vi "Demo.vi"() -> ()   [LabVIEW 2020, in "PowerControl.lvlib"]
uses:
  PowerControl.lvlib
  Labview Library/Libraries/Basic Experiment/CW settings.ctl
  YP03-60_X/YP03-60_X.lvclass
  C:/Labview Program/Labview_Control_SIC/Backup/VirtualPower/VirtualPower.lvclass
  YP03-60_Y/YP03-60_Y.lvclass
  YP03-60_Z/YP03-60_Z.lvclass
  VirtualPower/VirtualPower.lvclass
  Labview Library/Libraries/Basic Experiment/Basic Experiment.lvlib
panel:
  out "Pro":dbl[][](array[numeric])=[[-0.006013746913685614, -0.0005767508775091912, 0.003580211726197824, 0.002155800816019182, 0.0038511908961347263, 0.006438426694988175, -0.0017340280440567568, 0.005718743562201478, -0.004332868092551068, -0.00041017545622312745, -0.005538970864038539, -0.004012464200014998, -0.00792516643020258, -0.01574654474779913, -0.01310209587117428, -0.01651762842727922, -0.028081230793792877, -0.07887102008294333, -0.0966488744667412, -0.05726574286992636, -0.04009710278904244, -0.013943654119989213, -0.014891792267481052, -0.02856618593174698, -0.03385032526214127, -0.040599217504896146, -0.06044913845652411, -0.12219252863119912, -0.145572899201861, -0.12238330994007585, -0.07440755792421139, -0.04136503780617107, -0.03663431604289491, -0.022466284502222655, -0.009988690512261256, -0.007853472773907688, -0.0040597390725739535, -0.0010535701888517712, 0.001942673587738586, 0.0009046401382202252, -0.0022040602679889165], [0.00030942018483859357, 0.006545517163617287, -0.011571285455226787, -0.0005543704724179088, -0.00571613383603764, 0.003448168346978475, 0.0022478971389876534, -0.007040149065929868, 0.002513251653887716, 0.007368641761340111, 0.006313201433677307, -0.00947691386415117, -0.009153843171827547, -0.0012277679613130754, -0.009004290054349107, -0.022273516386379755, -0.04492940997686401, -0.07542469057166712, -0.10680439423841448, -0.06490179281471364, -0.043742806147826885, -0.03088586641820057, -0.03126158796986778, -0.03249904007682625, -0.04118533262413637, -0.06908010461555458, -0.10829568918119781, -0.1400238554264911, -0.10848703215017097, -0.06390484710798727, -0.03541632652309068, -0.019723273238761663, -0.017594711205418556, -0.01004862751091018, -0.00419887575862532, -0.011289191176208968, -0.003957013291320699, -0.00799541009422966, -0.005162780434214143, -0.006557950052931361, 0.00910905576244403], [0.006810636496503708, 0.010758157059567397, 0.00037187790202142246, -0.004975811124692475, -0.0022549265445015454, 0.004440990805914868, -0.005902149381657673, 0.0028450707010927445, -0.0013811589049794737, 0.005622914037517024, -0.007749721403714438, -0.011096664744028928, -0.006185456463094541, -0.014770720832796513, -0.006400699596351922, -0.01917068103315489, -0.03484291583179, -0.06696654295085125, -0.09429663190407978, -0.07022193366873686, -0.036127944880454343, -0.026433493814997933, -0.029596540512562775, -0.0547595204849165, -0.07934624397091083, -0.135303604851986, -0.14142779317873644, -0.11050981053166709, -0.05881398467255716, -0.042245426557882104, -0.02351994328283369, -0.019050385278118087, -0.009077854056939172, -0.007456997905022966, -0.004786728583101252, -0.01281291444557675, -0.0006758410166896045, -0.01320520210400744, 0.002038086253812299, 0.0057848989008100205, 0.0008845616357138208], [-0.002625712867039609, -0.0016672366841851138, 0.001523064957566156, 0.005031329580088562, 0.009562663666520255, -0.0133910818070474, 0.006351665826920705, -0.0032259111426599096, 0.002258900555879295, -0.001824194789903033, -0.010315416844289382, -0.014942445722062159, -0.010711646570336852, -0.008176873818602326, -0.0040919553812546194, -0.015920369318373595, -0.042856625587384456, -0.07552804437875049, -0.0974008995916611, -0.07697979712414382, -0.040526212336561174, -0.03947076513356085, -0.04879065588970799, -0.0785332509819675, -0.12130753027718966, -0.13003020401205556, -0.10267359275594912, -0.05305535890037516, -0.04023734109264043, -0.027311086417482477, -0.011703101371285607, -0.014214890568513328, -0.004168600486562424, -0.0038065115024557006, 0.003327740442873539, -0.004203702386747166, 0.0024552493679281806, 0.0029128960533322257, -0.0007063373708300347, -0.016710343019788576, 0.011280006287849531], [0.0027365602883753226, 0.005269264429016429, -0.0005940776192803199, 0.004109289952131778, 0.0030821311464996892, 0.0024789021275579692, -0.007451392313116756, -0.006446804599952394, -0.010433982385613993, -0.0052216141709899855, -0.0042187575181413806, -0.0024426611601837678, 0.0013822652502923916, -0.01472630714734835, -0.015310727619377906, -0.013700248199816967, -0.039748761113890474, -0.06000437633752398, -0.09049620162648231, -0.07708971572066847, -0.05175652860785329, -0.05510161667929925, -0.08047860025074871, -0.11699491465487777, -0.13342961820057853, -0.10648493059419517, -0.05852694394472624, -0.035506871113223704, -0.025867382420525997, -0.011268065661253046, -0.012128732558622346, -0.010910908366547956, -0.009326943407816701, -0.003980030193335038, -0.0029792182956402957, -0.005697697411583769, -0.006073014803772203, 0.004315543383023535, 0.004470928560230458, 0.001884290595045579, -0.0023510609586778752], [-0.0016149467898097791, 0.003866363318286714, 0.004551641770135451, -0.001287757308453541, -0.0015178735025507262, 0.0013606872198985709, -0.012437544484349194, -0.0042797764405111405, -0.002722577765502776, -0.0019964412861535052, -0.008832946243951367, 0.0033039456057690764, -0.010162356573933828, -0.010151076387070135, -0.019291417605513894, -0.02470984952515831, -0.024319474655931983, -0.042441505063211205, -0.0843977731248925, -0.09634700886930891, -0.0753659263040356, -0.06734873321330037, -0.10107364771887362, -0.13940536268000336, -0.11635069436014267, -0.0689028506053917, -0.02890616848972649, -0.028244135304359985, -0.014920328609911437, -0.014968727863628017, -0.008319724488920266, -0.01742963770347128, -0.0014620579322158767, -0.0058102156249267845, 0.004049482809928451, -0.010171769459133784, -0.0038191393595423673, -0.005824696341452884, 0.006530552298621428, 0.002148316863407551, -0.005279291552670484], [0.003018358685170197, 0.0007149998463948926, 0.008675189813975859, -0.0010138239232808655, -0.010883201638171691, -0.0023312340208446747, -0.008131024010790577, -0.00784879833945984, -0.0031996795159727753, -0.005437743050099142, 0.000672870043574747, -0.005897581602230972, -0.00872777599196406, -0.004103152270351629, -0.0024309124718483455, -0.015070473718634347, -0.017547412721379052, -0.036780820544978665, -0.06723032540015195, -0.10253914341445625, -0.07716073294286985, -0.087482309963969, -0.12634951791964522, -0.13230920186324302, -0.06885502128391052, -0.04309601026926624, -0.023394870549063085, -0.014664251602554357, -0.017079677295440576, -0.004779508059620574, -0.005344215558394261, -0.011358993782274895, -0.0033143187687716402, -0.004205847503612303, -0.003450640595654142, -0.0016550731991900047, -0.0022022307493323456, -0.00075512213292106, 0.0057207371279686114, -0.004223404191256663, -0.0023175273674425068], [0.0033744313398063053, 0.0057613604806578955, 0.00876360857579539, 0.0019871439832643834, 0.009537059189618224, -0.0035550699572037825, 0.004740524209693842, -0.0034764430161248194, -0.0033208036786522843, -0.005886710935717132, 0.0036394987717156546, 0.000562790249278855, -0.0012179574914809033, -0.009503429010038311, -0.0021131495169287584, -0.006498564982827637, -0.015687185644898682, -0.023057743862098357, -0.03817331807764324, -0.07651682008968097, -0.08614865177942743, -0.10949721630125442, -0.14223493346614635, -0.13448840732843725, -0.07173489757679907, -0.0407487167430064, -0.033220822786139026, -0.019565572158465883, -0.004030576210502845, -0.004985670737721826, -0.007339257072947136, -0.0098889248516707, -0.005704213866189911, -0.004179248206735986, -0.005170663370596684, -0.006431985576848431, -0.0006014895984396418, 0.0001401232558024823, -0.0031617286504207476, -0.0009844178298795692, 0.007752639724628807], [0.00020643963632838158, 0.0019652453346115095, -0.004693341193202527, 0.0025631545746047646, -0.002983259879286715, 0.0019373841691938676, 0.0026554242226808356, -0.0076405933254493075, -0.0011104967354892414, 0.00021186947118412292, 0.0043914003373171084, -0.014677264445715488, -0.004863640399563662, -0.0006246807569232349, -0.009017403176225458, -0.016771501001734412, -0.017913641675924907, -0.027922715397660225, -0.05637230985138064, -0.1053881611664782, -0.13951802336936547, -0.13536678420790016, -0.12130830776147905, -0.09727872340762045, -0.04740726934893158, -0.02771392653311222, -0.01794638844339358, -0.010568768611306845, -0.009219740541925758, -0.0010961352005850467, -0.002371173829414097, -0.0012811633460284577, -0.002790266973709654, -0.0042122498008142495, -0.00221145530027389, -0.003245753647569516, -0.00015469959712621772, -0.0016883723719409716, 0.01258460153950458, -0.0003041739758161688, -0.001895055258306244], [0.0025286594896174464, 0.007885085227719246, -0.0016720273103691952, 0.0021683975041422165, -0.0033329501977490406, -0.0006327507373690144, -0.0016032472842584244, -0.0015994025181752525, 9.146337248289171e-05, 0.006250846131687027, 0.00012262714951294384, -0.0030560550207286985, -0.009036847372346557, 0.0012033518840217639, -0.011192350096917103, -0.012198168738409398, -0.02162333146118356, -0.02157630700463886, -0.03548634090091274, -0.05826588763697027, -0.10181652762589477, -0.15475328527286614, -0.1347850176480042, -0.13008121677641482, -0.07505066119979065, -0.02823784475508817, -0.031131190269742204, -0.02269223620320826, -0.013333595621123573, -0.007881630914880255, 0.00182242613515049, 0.007606661616716082, 0.003534158261732756, 0.0075765896323594095, -0.004457376384760847, -0.002751068100449894, -0.0012253691521539878, 0.0037565041412528366, -0.004433340629326543, 0.0077859848518024855, -0.001037122546955871], [0.007378765083134731, 0.00461704029893073, -0.0004951575037919209, -0.001137325675469869, 0.0012670903202776085, -0.0073761685279288836, 0.013218324342143983, -0.01213133706843339, 0.0031377043940736815, -0.0013041111161846697, 0.00408381088001919, 0.008022737736488317, -0.013732613048574427, 0.0023411809508968595, -0.00834657652511761, -0.009682290606584765, -0.027120562654928237, -0.03155517647142092, -0.05488881595500106, -0.10399061567069867, -0.13452277720141126, -0.10987427852521259, -0.10520033655761696, -0.12692559344200982, -0.07615122751296965, -0.04250806118523409, -0.01863990933180537, -0.007932910868478471, -0.014960027791368291, 0.0006779428481562544, 0.0043326019972389496, 0.0012721191120537156, -0.00033225155340854684, -0.00459324948594253, -0.003763111674557451, 0.0014153182174410084, -0.00600875988629368, 0.002584711590019717, 0.000251267484822737, -0.0010910451377345032, 0.00434567429119892], [0.002607075511097845, 0.007268209395840941, -0.007143425461552666, -0.006842583851599082, -0.0017671515840863572, -0.0062626871548940866, 0.00743625608616183, -0.002280314918964188, -0.007790886195496283, 0.0009045175985771259, -0.0004795588642588777, -0.0022580913534406832, -0.006557058858322584, -0.002918677905747402, -0.005883932815465842, -0.014976878538155214, -0.007953039857539146, -0.011378460757218933, -0.030689087614390487, -0.07209631629090507, -0.11103251751760701, -0.1274402994442292, -0.09171277858124949, -0.09286719137449906, -0.1070560647507438, -0.06948372772366862, -0.03625772950992301, -0.026947559988784286, -0.01775673449630233, -0.007092102210007334, -0.01462269459622012, -0.0011244478595424656, -0.010959113619225413, -0.004203351715154291, -0.010840958515320742, 0.00019376873199861144, 0.0025871407298798665, -0.011068023804326144, 0.0010563936346741354, 0.0017343783704297788, -0.005973830269607183], [0.0010717602931125114, 0.0004781479000275368, 0.00106403873281824, -0.010476325577616352, 0.0024755833150873485, 0.0005481859560085844, -0.0014467519986510746, 0.0040609761279231105, 0.004709079447832387, -0.0024612223992098725, 0.009130479666112468, 0.0036674759984731686, 0.006410491379179817, -0.0014389986985525738, -0.005734939448449161, 0.002862492594718713, -0.004771634257221047, -0.02597886046152098, -0.026981178786879667, -0.04144669393406386, -0.0844950151592414, -0.12157619962651134, -0.09517743780643517, -0.06904199028502112, -0.06658716906415874, -0.09686649532539793, -0.06241426203625822, -0.04219380713878684, -0.018237447050885036, -0.016307991950545442, -0.012442846242940675, -0.014649694658002033, -0.008787655832126484, 0.0018914236460587652, 0.005545868561422029, -0.0038691097583342104, -0.001782181609653044, 0.013593888688889555, -0.004041841643779187, 0.005652503330171976, -0.0017965849029641934]]
  in  "Direction":enum16{"X", "Y", "Z"}(ring)
  out "Result":dbl[][](array[numeric])=[[1358.1087120306884, 1347.8140053880857], [1357.008056458632, 1347.8808631501881], [1355.8138681934734, 1347.9001189162352], [1354.8413881609904, 1347.892976344908], [1353.913391643344, 1348.0718328974717], [1353.2442149475337, 1348.616017834578], [1352.5498698485417, 1348.8747670873547], [1351.9182726681042, nan], [1350.0708234254153, 1352.1304648799637], [1351.0759709104414, 1352.6920411960402], [1349.8173117381086, 1352.8864528821034], [1350.6127202130124, 1353.9867592118412], [1351.0334561831235, 1355.2380696382204]]
  in  "Settings":T1={"Num Pts"=50, "Start freq"=1320.0, "Stop freq"=1400.0, " dBm"=-16.0, "Ratio \nThre(abs)"=0.06, "AutoTrace Before Exp"=TRUE, "RepoSave"=FALSE, "Peak Num \nLimit "=2, "Loop per Update"=1000, "UpdateTime"=40} {"UpdateTime" format="%.0p"; "Loop per Update" format="%#_6p"}
  in  "Num":i32
  in  "CurrentMax(X)":dbl
  in  "CurrentMin(X)":dbl
  in  "VISA resource name":refnum<visa-resource-name>
  in  "Current(0)":dbl
  # "CW Settings"
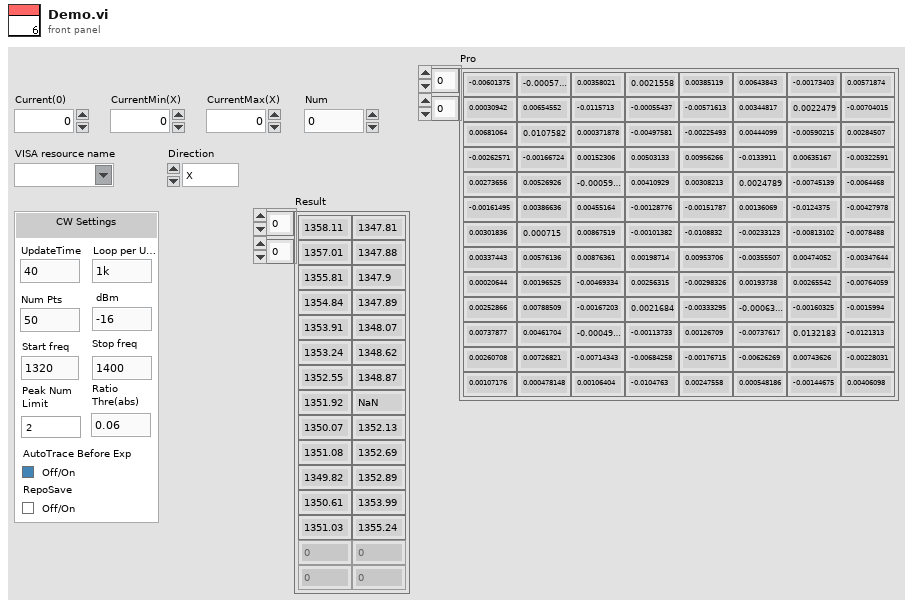
[diagram p1: front panel]
types:
  T1 = typedef "Basic Experiment.lvlib/CW settings.ctl" = cluster{"Num Pts":i32, "Start freq":dbl, "Stop freq":dbl, " dBm":dbl, "Ratio \nThre(abs)":dbl, "AutoTrace Before Exp":bool, "RepoSave":bool, "Peak Num \nLimit ":i32, "Loop per Update":u32, "UpdateTime":i32}
  T2 = typedef "Basic Experiment.lvlib/CW Results.ctl" = cluster{"Fit Frequency":T3, "Pro":dbl[], "Error Bar":dbl[], "Raw Data Path":path, "Image Path":path}
  T3 = typedef "Basic Experiment.lvlib/CW Fit Frequency.ctl" = cluster{"Fre2":cluster{"Amplitude":dbl, "Position":dbl, "Width":dbl}, "Fre1":cluster{"Amplitude":dbl, "Position":dbl, "Width":dbl}, "Fre3":cluster{"Amplitude":dbl, "Position":dbl, "Width":dbl}, "Background":dbl}
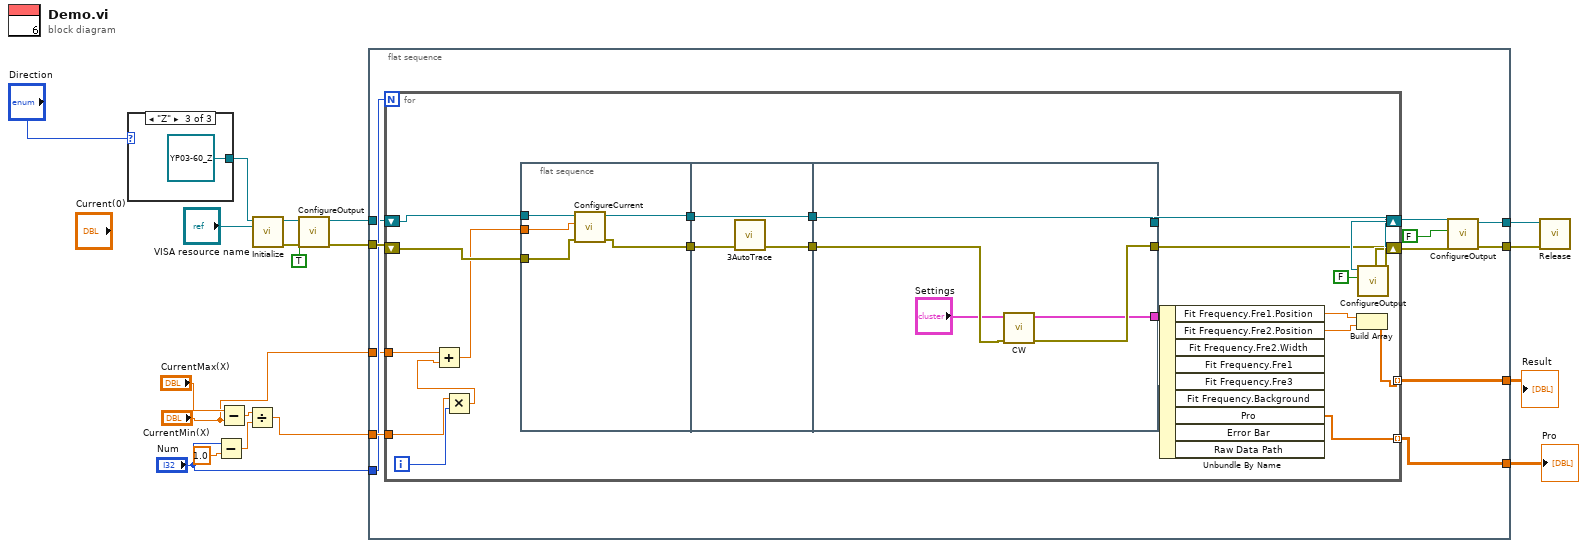
[diagram p0: block diagram]
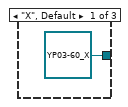
[diagram p2: hidden frame]
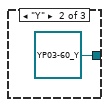
[diagram p3: hidden frame]
diagram:
  n1 = case shown="\"Z\"" "Direction" {
    tunnel: [refnum<class "YP03-60_X.lvclass"> refnum ("PowerControl.lvlib:YP03-60_X.lvclass") refnum<class "YP03-60_Y.lvclass"> refnum ("PowerControl.lvlib:YP03-60_Y.lvclass") refnum<class "YP03-60_Z.lvclass"> refnum ("PowerControl.lvlib:YP03-60_Z.lvclass")] -> w6
    frame "X", Default {
    }
    frame "Y" {
    }
    frame "Z" {
    }
  }
  n2 = Subtract(x="Num", y=1.0) -> (x-y=w11:dbl)
  n3 = Subtract(x="CurrentMax(X)", y="CurrentMin(X)") -> (x-y=w14:dbl)
  n4 = Divide(x=w14, y=w11) -> (x/y=w13:dbl)
  n5 = call-dynamic "Initialize.vi"("VISA resource name"="VISA resource name", "VirtualPower in"=w6) -> ("error out"=w17:errorcluster, "VirtualPower out"=w18:refnum<class "VirtualPower.lvclass">)  [unwired: 8 in]
  n6 = call-dynamic "ConfigureOutput.vi"("error in (no error)"=w17, "Output((F)"=TRUE, "VirtualPower in"=w18) -> ("error out"=w16:errorcluster, "VirtualPower out"=w5:refnum<class "VirtualPower.lvclass">)  [unwired: 7 in]
  n7 = flat-sequence {
    tunnel: w16 -> [w33]
    tunnel: w13 -> [w32]
    tunnel: "Num" -> [w31]
    tunnel: [w30] -> w8
    tunnel: w5 -> [w29]
    tunnel: [w28] -> w4
    tunnel: [w26] -> w3
    tunnel: "CurrentMin(X)" -> [w24]
    tunnel: [w23] -> w1
    frame #0 {
      n8 = for {
        N: w31 -> [_]
        shift-right: [w54] -> w35
        shift-left: w29 -> [w52]
        shift-right: [w53] -> w34
        shift-left: w33 -> [w55]
        tunnel: w32 -> [w51]
        tunnel: [w42] -> w30 mode=indexing
        tunnel: w24 -> [w39]
        tunnel: [w38] -> w23 mode=indexing
        i -> [w50]
        n9 = Multiply(x=w51, y=w50) -> (x*y=w40:dbl)
        n10 = Add(x=w39, y=w40) -> (x+y=w41:dbl)
        n11 = flat-sequence {
          tunnel: w55 -> [w58]
          tunnel: [w59] -> w48
          tunnel: [w57] -> w46
          tunnel: w52 -> [w60]
          tunnel: w41 -> [w56]
          tunnel: w48 -> [w63]
          tunnel: [w63] -> w47
          tunnel: w46 -> [w62]
          tunnel: [w61] -> w45
          tunnel: [w66] -> w53
          tunnel: [w68] -> w54
          tunnel: w47 -> [w68]
          tunnel: [w65] -> w49
          tunnel: w45 -> [w67]
          frame #0 {
            n12 = call-dynamic "ConfigureCurrent.vi"("error in (no error)"=w58, "Current(0)"=w56, "VirtualPower in"=w60) -> ("error out"=w57:errorcluster, "VirtualPower out"=w59:refnum<class "VirtualPower.lvclass">)  [unwired: 7 in]
          }
          frame #1 {
            n13 = call "3AutoTrace.vi"("error in"=w62) -> ("error out"=w61:errorcluster)  [unwired: 6 in, 2 out]
          }
          frame #2 {
            n14 = call "CW.vi"("error in (no error)"=w67, "Settings"="Settings") -> ("error out"=w66:errorcluster, "CW Result"=w65:T2)  [unwired: 7 in, 1 out]
          }
        }
        n15 = Unbundle By Name(w49) -> ("Fit Frequency.Fre1.Position"=w44:dbl, "Fit Frequency.Fre2.Position"=w43:dbl, "Pro"=w38:dbl[])  [unwired: 6 out]
        n16 = Build Array(w44, w43) -> (w42:dbl[])
      }
      n17 = call-dynamic "ConfigureOutput.vi"("error in (no error)"=w34, "Output((F)"=FALSE, "VirtualPower in"=w35) -> ("error out"=w36:errorcluster, "VirtualPower out"=w27:refnum<class "VirtualPower.lvclass">)  [unwired: 7 in]
      n18 = call-dynamic "ConfigureOutput.vi"("error in (no error)"=w36, "Output((F)"=FALSE, "VirtualPower in"=w27) -> ("error out"=w28:errorcluster, "VirtualPower out"=w26:refnum<class "VirtualPower.lvclass">)  [unwired: 7 in]
    }
  }
  n19 = call-dynamic "Release.vi"("error in (no error)"=w4, "VirtualPower in"=w3) -> ()  [unwired: 9 in, 1 out]
  "Result" <- w8
  "Pro" <- w1
